vi "HEI_CTRL.vi"(8 "shutdown":i32, 9 "Set RPM":i32, 10 "Remote / Manual":bool, 11 "port3":i32) -> ()   [LabVIEW 2017]
uses:
  BERTTA.dll
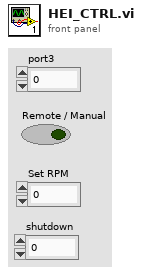
[diagram p1: front panel]
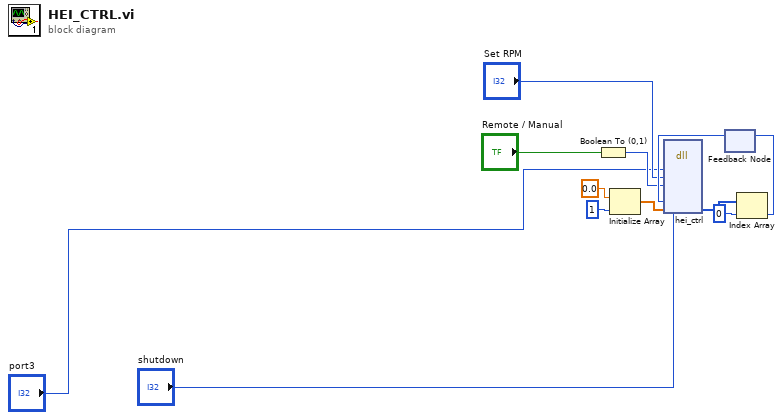
[diagram p0: block diagram]
diagram:
  n1 = Boolean To (0,1)(Boolean="Remote / Manual") -> (0, 1=w4:i16)
  n2 = Initialize Array(0.0 ("element"), 1 ("dimension size")) -> (w7:dbl[])
  n3 = feedback #1() -> (w11:i32)  [unwired: 1 in]
  n4 = dll-call lib="C:/Users/shresplab/OneDrive - Kemira Oyj/Documents/GitHub/Bertta/BERTTA/x64/Debug/BERTTA.dll" fn="hei_ctrl"("port"="port3", "speed"="Set RPM", "manual"=w4, "shutdown"="shutdown", "prev_status"=w11, "status"=w7) -> ("status"=w6:i32[])  [unwired: 9 in, 2 out]
  n5 = Index Array(array=w6, index=0) -> (element=w10:i32)
  n6 = feedback-in #1(w10) -> ()
